vi "Extract Lines on Grass temp.vi"() -> ()   [LabVIEW 2009]
doc: "VI which takes an image and outputs marked regions. One for the left and one for the right"
uses:
  <vilib>/vision/Image Controls.llb/IMAQ Image.ctl
  <vilib>/vision/NI_Vision_Development_Module.lvlib
panel:
  out "Image Dst Out":T1(plugin-control)
  out "Image Out":T1
  out "Number of Particles1":i32
  out "error out":errorcluster
  out "Number of Particles":i32
  in  "error in (no error)":errorcluster
  out "Original":T1(plugin-control)
  in  "File Path":path
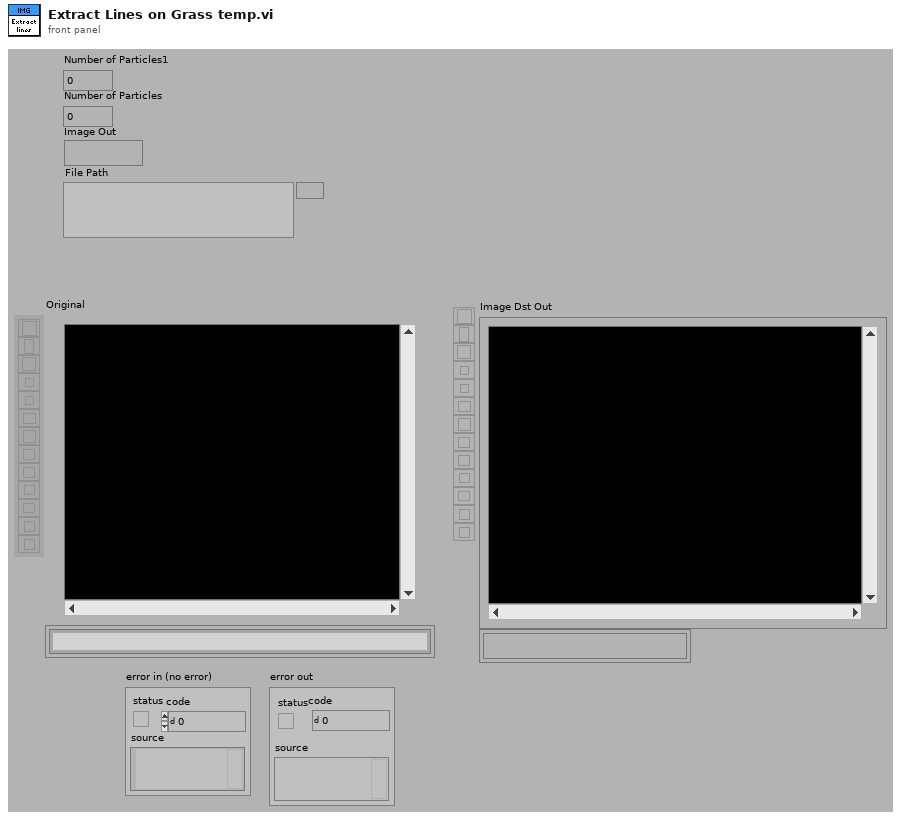
[diagram p1: front panel]
types:
  T1 = typedef "IMAQ Image.ctl" = refnum<image>
  T2 = typedef "Image Type" = u32
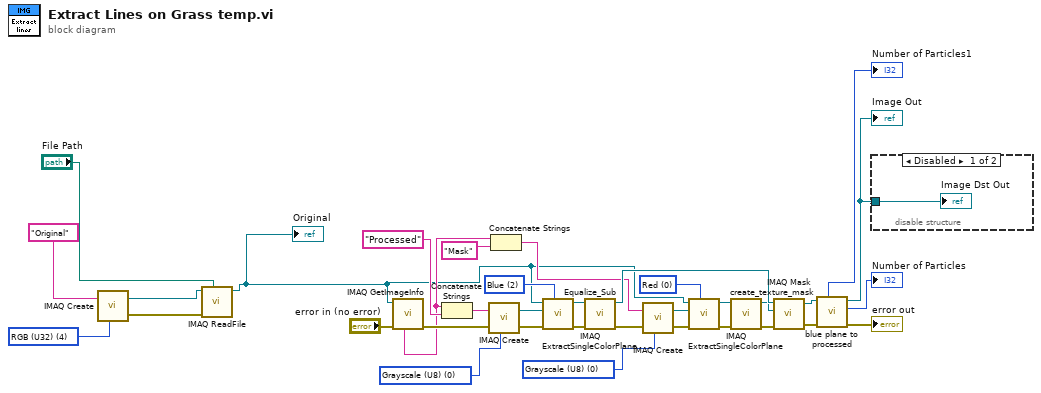
[diagram p0: block diagram]
diagram:
  w18 = T2 0 items=["Grayscale (U8)", "Grayscale (I16)", "Grayscale (SGL)", "Complex (CSG)", "RGB (U32)", "HSL (U32)", "RGB (U64)"] ("Image Type")
  w21 = 0 items=["Red", "Green", "Blue", "Hue", "Saturation", "Luminance", "Value", "Intensity"] ("Color Plane")
  w25 = 2 items=["Red", "Green", "Blue", "Hue", "Saturation", "Luminance", "Value", "Intensity"] ("Color Plane")
  w28 = T2 0 items=["Grayscale (U8)", "Grayscale (I16)", "Grayscale (SGL)", "Complex (CSG)", "RGB (U32)", "HSL (U32)", "RGB (U64)"] ("Image Type")
  w33 = T2 4 items=["Grayscale (U8)", "Grayscale (I16)", "Grayscale (SGL)", "Complex (CSG)", "RGB (U32)", "HSL (U32)", "RGB (U64)", "Grayscale (U16)"] ("Image Type")
  n1 = call "IMAQ Create"("Image Name"="Original", "Image Type"=w33) -> ("New Image"=w31:T1, "error out"=w35:errorcluster)  [unwired: 3 in]
  n2 = call "IMAQ ReadFile"("File Path"="File Path", "error in (no error)"=w35, "Image"=w31) -> ("Image Out"=w1:T1)  [unwired: 4 in, 4 out]
  "Original" <- w1
  n3 = call "IMAQ GetImageInfo"("error in (no error)"="error in (no error)", "Image"=w1) -> ("error out"=w10:errorcluster, "Image Name"=w5:string)  [unwired: 8 out]
  n4 = Concatenate Strings(w5, "Processed" ("Image Name")) -> (w7:string)
  n5 = call "IMAQ Create"("Image Name"=w7, "Image Type"=w18, "error in (no error)"=w10) -> ("New Image"=w20:T1, "error out"=w19:errorcluster)  [unwired: 1 in, 1 out]
  n6 = Concatenate Strings(w5, "Mask" ("Image Name")) -> (w8:string)
  n7 = call "IMAQ ExtractSingleColorPlane"("Color Plane"=w25, "error in (no error)"=w19, "Image Dst"=w20, "Image Src"=w1) -> ("error out"=w24:errorcluster, "Image Dst Out"=w23:T1)  [unwired: 6 out]
  n8 = call "Equalize_Sub.vi"("error in (no error)"=w24, "Image Src"=w23) -> ("error out"=w27:errorcluster, "Image Out"=w30:T1)  [unwired: 8 out]
  n9 = call "IMAQ Create"("Image Name"=w8, "Image Type"=w28, "error in (no error)"=w27) -> ("New Image"=w17:T1, "error out"=w22:errorcluster)  [unwired: 1 in, 1 out]
  n10 = call "IMAQ ExtractSingleColorPlane"("Color Plane"=w21, "error in (no error)"=w22, "Image Dst"=w17, "Image Src"=w1) -> ("error out"=w16:errorcluster, "Image Dst Out"=w12:T1)  [unwired: 6 out]
  n11 = call "create_texture_mask.vi"("error in (no error)"=w16, "Image Src"=w12) -> ("error out"=w29:errorcluster, "Image"=w26:T1)  [unwired: 8 out]
  n12 = call "IMAQ Mask"("error in (no error)"=w29, "Image Mask"=w26, "Image Src"=w30) -> ("error out"=w14:errorcluster, "Image Dst Out"=w15:T1)  [unwired: 1 in, 1 out]
  n13 = call "blue plane to processed.vi"("error in (no error)"=w14, "Image Src"=w15) -> ("error out"=→"error out":errorcluster, "Number of Particles"=→"Number of Particles":i32, "Image Dst Out"=w2:T1, "Number of Particles1"=→"Number of Particles1":i32)  [unwired: 6 out]
  "Image Out" <- w2
  n14 = disable-structure shown="Disabled" {
    disable-tunnel: w2 -> [w36 _]
    frame #0 {
      "Image Dst Out" <- w36
    }
    frame #1 {
    }
  }
